vi "GetText.vi"(8 "error in":errorcluster, 11 "OPC UA editor node in":refnum<class "OPC UA Client editor node.lvclass">) -> (0 "error out":errorcluster, 1 "additional text":string, 2 "text":string, 3 "OPC UA editor node out":refnum<class "OPC UA Client editor node.lvclass">, 4 "glyph":string)   [LabVIEW 2014, in "OPC UA Client editor node.lvclass"]
uses:
  OPC UA Client editor node.lvclass
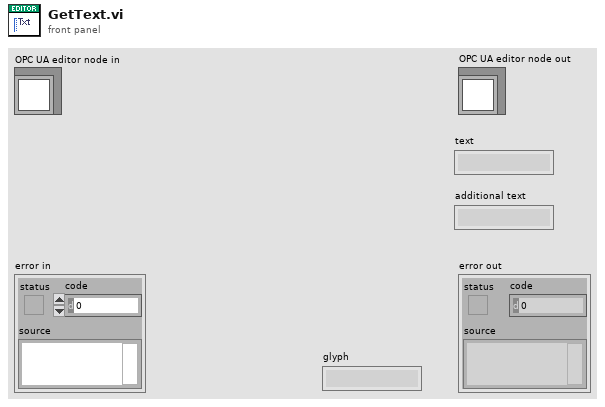
[diagram p1: front panel]
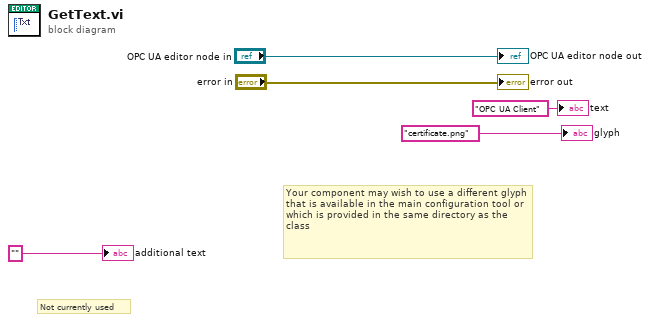
[diagram p0: block diagram]
diagram:
  # "Not currently used"
  # "Your component may wish to use a different glyph that is available in the main configuration tool or which is provided in the same directory as the class"
  "error out" <- "error in"
  "OPC UA editor node out" <- "OPC UA editor node in"
  "text" <- "OPC UA Client" ("text")
  "additional text" <- "" ("additional text")
  "glyph" <- "certificate.png" ("glyph")
